vi "remove one element in array.vi"(7 "element to remove":dbl, 11 "Input":dbl[](array[numeric])) -> (3 "Output":dbl[](array[numeric]))   [LabVIEW 2023]
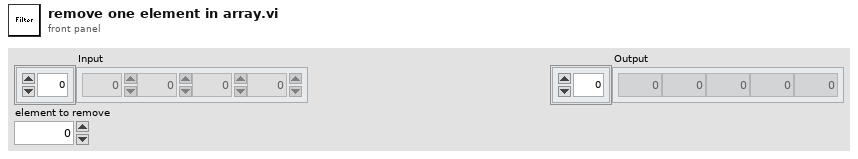
[diagram p1: front panel]
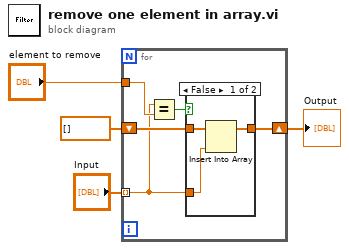
[diagram p0: block diagram]
diagram:
  n1 = for {
    tunnel: "Input" -> [w5] mode=indexing
    tunnel: "element to remove" -> [w9]
    shift-right: [w6] -> w1
    shift-left: dbl[] [] ("array") -> [w7]
    n2 = Equal?(x=w5, y=w9) -> (x = y?=w8:bool)
    n3 = case shown="False" w8 {
      tunnel: w7 -> [w12 w13]
      tunnel: [w10 w13] -> w6
      tunnel: w5 -> [w11 _]
      frame False {
        n4 = Insert Into Array(array=w12, new element=w11) -> (w10:dbl[])  [unwired: 1 in]
      }
      frame True {
      }
    }
  }
  "Output" <- w1
